vi "UE9 Stream AIN with Timers & Counters.vi"() -> ()   [LabVIEW 2021]
panel:
  in  "Reset Timer1/Counter0":bool
  out "Combined Counter Data":u32[](array[numeric])
  out "Comm Backlog":i32
  out "# Scans Read":i32
  out "# of iterations":i32
  out "Data":dbl[][](array[numeric]) format="%.3f"
  in  "Scan Rate (Hz)":dbl=1000.0 format="%.3f"
  in  "FirstFound":bool=TRUE
  in  "stop":bool
  in  "ConnectionType":u16(ring) items=["LJ_ctUSB", "LJ_ctETHERNET"]
  in  "DeviceType":u16(ring)=1 items=["LJ_dtU3", "LJ_dtUE9"]
  in  "Address":string="192.168.1.209"
  out "Error Message":string
  # "This example streams AIN0, Timer1 (duty cycle input on\nFIO1), Counter0 (FIO2), and the FIO/EIO digital inputs.\n\nTimer0 is configured as 16-bit PWM output (FIO0).  Frequency\nis 40.6 Hz and duty cycle is 25%.\n\nFor testing, short FIO0 to FIO1 and FIO2."
  # "AIN0               TMR1 (LSW)         TMR1 (MSW)    CNT (LSW)        CNT(MSW)        FIO/EIO"
  # "Specify an IP address for Ethernet, or\nLocal ID for USB.  If FirstFound is selected,\nLocal ID is ignored for USB.  Clear\nFirstFound if using Ethernet."
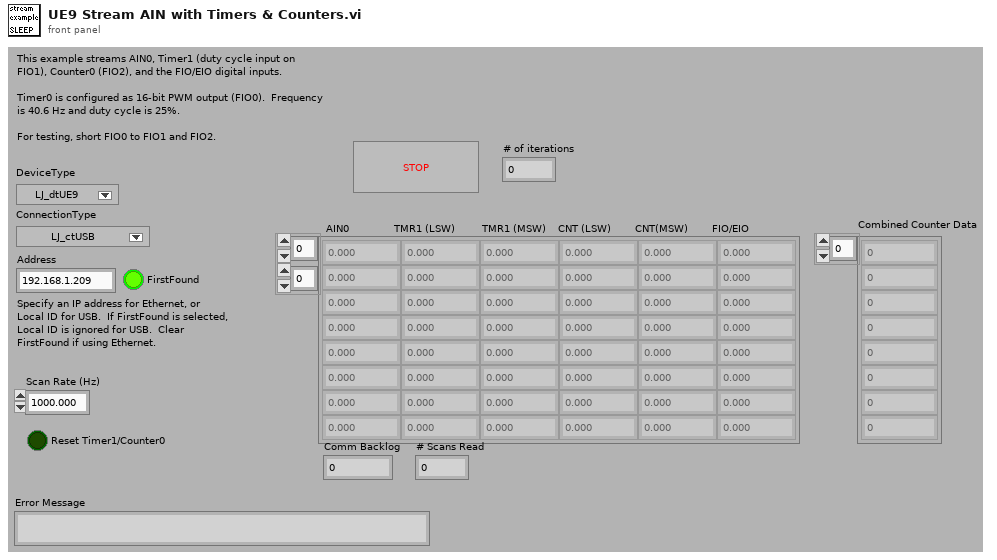
[diagram p1: front panel]
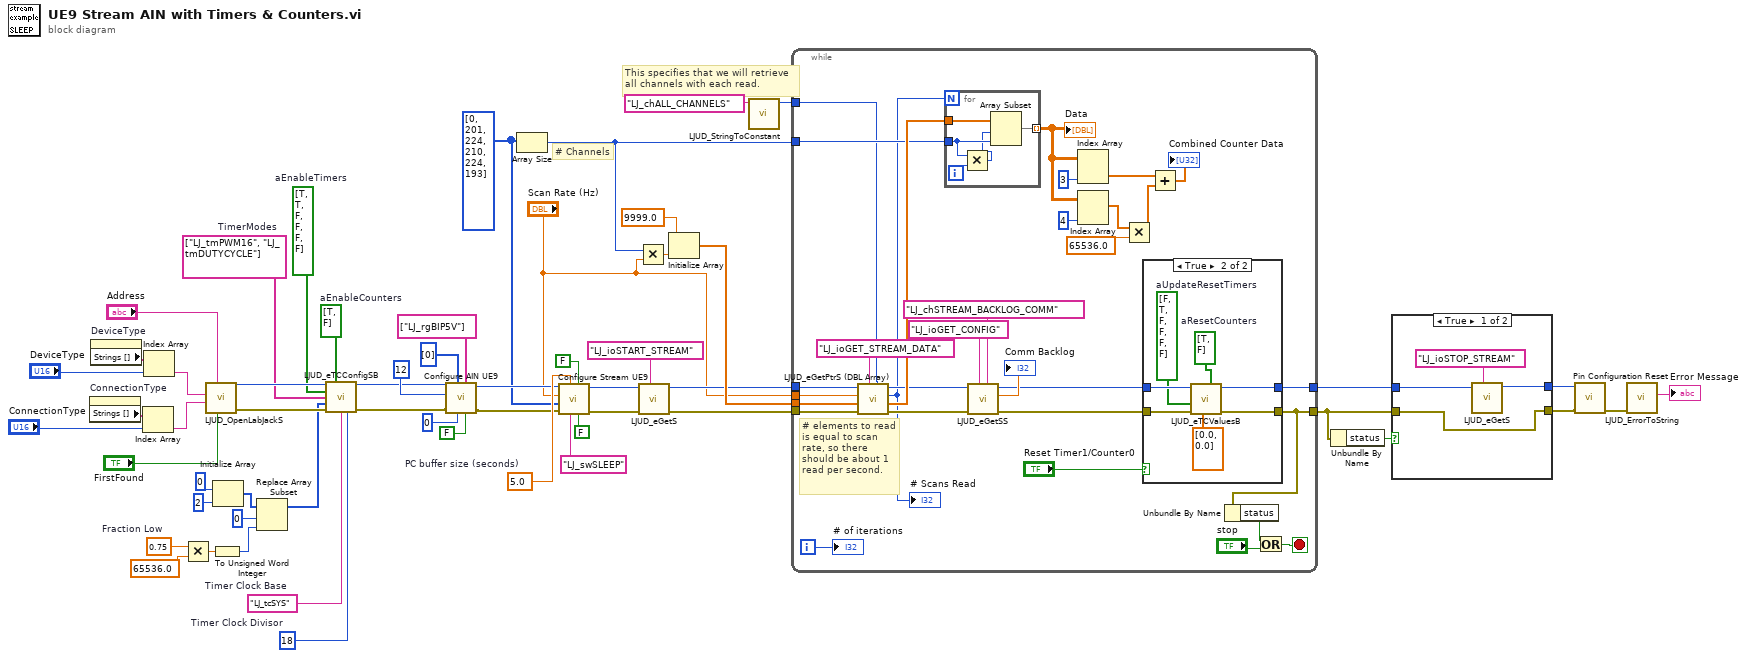
[diagram p0: block diagram]
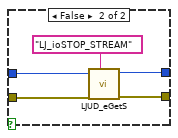
[diagram p3: hidden frame]
diagram:
  w4 = 18  # Timer Clock Divisor
  w5 = "LJ_tcSYS"  # Timer Clock Base
  w8 = bool[] [TRUE, FALSE]  # aEnableCounters
  w10 = 0.75  # Fraction Low
  w6 = string[] ["LJ_tmPWM16", "LJ_tmDUTYCYCLE"]  # TimerModes
  w7 = bool[] [TRUE, TRUE, FALSE, FALSE, FALSE, FALSE]  # aEnableTimers
  w22 = i32[] [0, 201, 224, 210, 224, 193] ("Channels")
  w44 = 5.0  # PC buffer size (seconds)
  # "# Channels"
  # "This specifies that we will retrieve\nall channels with each read."
  n1 = property on="ConnectionType" class="Ring (strict)"() -> ("Strings []"=w36:string[])  [unwired: 2 in, 2 out]
  n2 = property on="DeviceType" class="Ring (strict)"() -> ("Strings []"=w37:string[])  [unwired: 2 in, 2 out]
  n3 = Index Array(array=w36, index="ConnectionType") -> (element=w32:string)
  n4 = Index Array(array=w37, index="DeviceType") -> (element=w33:string)
  n5 = Multiply(x=w10, y=65536.0) -> (x*y=w12:dbl)
  n6 = call "LJUD_OpenLabJackS.vi"("FirstFound"="FirstFound", "Address"="Address", "ConnectionType"=w32, "DeviceType"=w33) -> ("error out"=w18:errorcluster, "Handle"=w19:i32)  [unwired: 5 in, 1 out]
  n7 = To Unsigned Word Integer(number=w12) -> (unsigned 16bit integer=w11:u16)
  n8 = Initialize Array(u16 0 ("PWM Timer Value"), 2 ("Dimension Size")) -> (w14:u16[])
  n9 = Replace Array Subset(array=w14, new element=w11, index=0 ("Index")) -> (w9:u16[])
  n10 = call "LJUD_eTCConfigSB.vi"("Handle In"=w19, "aEnableCounters"=w8, "aEnableTimers"=w7, "aTimerModes"=w6, "aTimerValues"=w9, "error in"=w18, "TimerClockBase"=w5, "TimerClockDivisor"=w4) -> ("Handle Out"=w21:i32, "error out"=w20:errorcluster)  [unwired: 6 in]
  n11 = call "Configure AIN UE9.vi"("Binary"=FALSE, "Ranges"=string[] ["LJ_rgBIP5V"], "SettlingFactor"=0, "Channels"=i32[] [0], "error in"=w20, "Resolution"=12, "Handle In"=w21) -> ("error out"=w41:errorcluster, "Handle Out"=w40:i32)  [unwired: 3 in]
  n12 = Array Size(array=w22) -> (size(s)=w48:i32)
  n13 = call "Configure Stream UE9.vi"("External Scan Trigger"=FALSE, "Scan Clock Output"=FALSE, "Wait Mode"="LJ_swSLEEP" ("Wait Mode (2)"), "PC buffer size (seconds)"=w44, "error in"=w41, "Scan List"=w22, "Scan Rate (Hz)"="Scan Rate (Hz)", "Handle In"=w40) -> ("error out"=w53:errorcluster, "Handle Out"=w54:i32)  [unwired: 1 in, 1 out]
  n14 = Multiply(x=w48, y="Scan Rate (Hz)") -> (x*y=w51:dbl)
  n15 = call "LJUD_eGetS.vi"("IOType"="LJ_ioSTART_STREAM", "error in"=w53, "Handle In"=w54) -> ("error out"=w52:errorcluster, "Handle Out"=w39:i32)  [unwired: 6 in, 1 out]
  n16 = Initialize Array(9999.0, w51) -> (w49:dbl[])
  n17 = call "LJUD_StringToConstant.vi"("String"="LJ_chALL_CHANNELS") -> ("Constant Number"=w28:i32)  [unwired: 9 in, 1 out]
  n18 = while {
    tunnel: w28 -> [w73]
    tunnel: [w60] -> w31
    tunnel: [w59] -> w46
    tunnel: w48 -> [w80]
    tunnel: w49 -> [w83]
    tunnel: "Scan Rate (Hz)" -> [w81]
    tunnel: w52 -> [w85]
    tunnel: w39 -> [w86]
    i -> [w79]
    stop <- w72 stop-if-true
    # "# elements to read\nis equal to scan\nrate, so there\nshould be about 1\nread per second."
    n19 = call "LJUD_eGetPtrS (DBL Array).vi"("Channel"=w73, "IOType"="LJ_ioGET_STREAM_DATA", "error in"=w85, "DBL Array Write"=w83, "Value"=w81, "Handle In"=w86) -> ("error out"=w77:errorcluster, "DBL Array Read"=w82:dbl[], "Value"=w71:i32, "Handle Out"=w78:i32)  [unwired: 2 in]
    "# Scans Read" <- w71
    n20 = for {
      N: w71 -> [_]
      tunnel: w82 -> [w102]
      tunnel: w80 -> [w101]
      tunnel: [w98] -> w70 mode=indexing
      i -> [w100]
      n21 = Multiply(x=w101, y=w100) -> (x*y=w99:i32)
      n22 = Array Subset(array=w102, index=w99, length=w101) -> (w98:dbl[])
    }
    "Data" <- w70
    n23 = call "LJUD_eGetSS.vi"("Channel"="LJ_chSTREAM_BACKLOG_COMM", "IOType"="LJ_ioGET_CONFIG", "error in"=w77, "Handle In"=w78) -> ("error out"=w62:errorcluster, "Value Read"=→"Comm Backlog":dbl, "Handle Out"=w61:i32)  [unwired: 5 in]
    n24 = Index Array(array=w70, index (col)=3 ("Disabled Index (col)")) -> (element=w66:dbl[])  [unwired: 1 in]
    n25 = Index Array(array=w70, index (col)=4 ("Disabled Index (col)")) -> (element=w67:dbl[])  [unwired: 1 in]
    n26 = Multiply(x=w67, y=65536.0) -> (x*y=w65:dbl[])
    n27 = case shown="True" "Reset Timer1/Counter0" {
      tunnel: w62 -> [w90 w97]
      tunnel: w61 -> [w89 w96]
      tunnel: [w90 w95] -> w60
      tunnel: [w89 w94] -> w59
      frame False {
      }
      frame True {
        w93 = bool[] [TRUE, FALSE]  # aResetCounters
        w92 = bool[] [FALSE, TRUE, FALSE, FALSE, FALSE, FALSE]  # aUpdateResetTimers
        n28 = call "LJUD_eTCValuesB.vi"("aResetCounters"=w93, "aTimerValues Write"=dbl[] [0.0, 0.0], "error in"=w97, "aUpdateResetTimers"=w92, "Handle In"=w96) -> ("error out"=w95:errorcluster, "Handle Out"=w94:i32)  [unwired: 3 in, 2 out]
      }
    }
    n29 = Add(x=w66, y=w65) -> (x+y=→"Combined Counter Data":dbl[])
    n30 = Unbundle By Name(w60) -> ("status"=w87:bool)
    n31 = Or(x=w87, y="stop") -> (x .or. y?=w72:bool)
    "# of iterations" <- w79
  }
  n32 = Unbundle By Name(w31) -> ("status"=w30:bool)
  n33 = case shown="True" w30 {
    tunnel: w46 -> [w105 w110]
    tunnel: [w104 w109] -> w3
    tunnel: w31 -> [w104 w108]
    tunnel: [w103 w107] -> w1
    frame True {
      n34 = call "LJUD_eGetS.vi"("IOType"="LJ_ioSTOP_STREAM", "Handle In"=w105) -> ("Handle Out"=w103:i32)  [unwired: 7 in, 2 out]
    }
    frame False {
      n35 = call "LJUD_eGetS.vi"("IOType"="LJ_ioSTOP_STREAM", "error in"=w108, "Handle In"=w110) -> ("error out"=w109:errorcluster, "Handle Out"=w107:i32)  [unwired: 6 in, 1 out]
    }
  }
  n36 = call "Pin Configuration Reset.vi"("error in"=w3, "Handle In"=w1) -> ("error out"=w2:errorcluster)  [unwired: 8 in, 1 out]
  n37 = call "LJUD_ErrorToString.vi"("error in"=w2) -> ("String"=→"Error Message":string)  [unwired: 10 in]
